vi "Pack A0 Values.vi"(9 "AO Values":dbl[](array[numeric]), 10 "AO Resolution (Bits)":u8, 11 "Analog Ref Override":dbl) -> (3 "Packet Values":u8[](array[numeric]) format="%.0b")   [LabVIEW 2020, in "Device.lvlib"]
uses:
  Device.lvlib
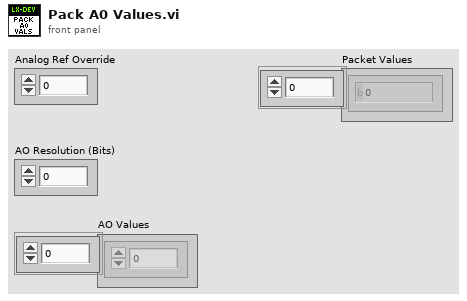
[diagram p1: front panel]
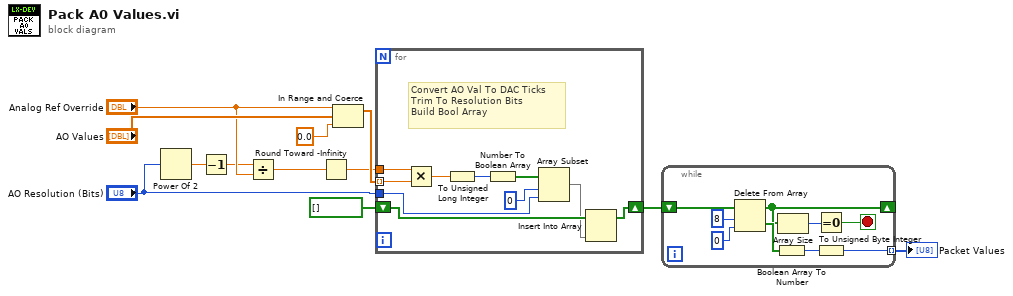
[diagram p0: block diagram]
diagram:
  n1 = Power Of 2(x="AO Resolution (Bits)") -> (2^x=w7:dbl)
  n2 = Decrement(x=w7) -> (x-1=w6:dbl)
  n3 = Divide(x=w6, y="Analog Ref Override") -> (x/y=w5:dbl)
  n4 = Round Toward -Infinity(1:w5) -> (0:w4:dbl)
  n5 = In Range and Coerce(upper limit="Analog Ref Override", x="AO Values", lower limit=0.0 ("AI Ref (V)")) -> (coerced(x)=w10:dbl[])  [unwired: 1 out]
  n6 = for {
    tunnel: w10 -> [w21] mode=indexing
    tunnel: w4 -> [w22]
    tunnel: "AO Resolution (Bits)" -> [w16]
    shift-right: [w13] -> w2
    shift-left: bool[] [] -> [w15]
    # "Convert AO Val To DAC Ticks\nTrim To Resolution Bits\nBuild Bool Array"
    n7 = Multiply(x=w22, y=w21) -> (x*y=w20:dbl)
    n8 = To Unsigned Long Integer(number=w20) -> (unsigned 32bit integer=w19:u32)
    n9 = Number To Boolean Array(number=w19) -> (Boolean array=w18:bool[])
    n10 = Array Subset(array=w18, index=0, length=w16) -> (w14:bool[])
    n11 = Insert Into Array(array=w15, new element=w14) -> (w13:bool[])  [unwired: 1 in]
  }
  n12 = while {
    shift-right: [w26] -> _
    shift-left: w2 -> [w31]
    tunnel: [w27] -> w1 mode=indexing
    stop <- w24 stop-if-true
    n13 = Delete From Array(array=w31, length=8, index=0) -> (deleted portion=w29:bool[], array with subset deleted=w26:bool[])
    n14 = Boolean Array To Number(Boolean array=w29) -> (number=w28:u32)
    n15 = Array Size(array=w26) -> (size(s)=w25:i32)
    n16 = Equal To 0?(x=w25) -> (x = 0?=w24:bool)
    n17 = To Unsigned Byte Integer(number=w28) -> (unsigned 8bit integer=w27:u8)
  }
  "Packet Values" <- w1
